vi "Configure OVP.vi"(7 "Enable OVP (T: Enable)":bool=TRUE, 8 "error in (no error)":errorcluster, 9 "Voltage Limit (6.5 V)":dbl=6.5 format="%.2f", 10 "Channel (0: 30V Channel)":T1 caption="Channel (0: +6V)" items=["30V/3A Channel", "30V/3A Channel", "5V/3A Channel"], 11 "VISA resource name":refnum<visa-resource-name>) -> (0 "error out":errorcluster, 3 "VISA resource name out":refnum<visa-resource-name>)   [LabVIEW 2020, in "RIGOL DP800 Series.lvlib"]
doc: "Configures over voltage protection (OVP) of the power supply. Specify the voltage limit and whether to enable or disable OVP."
uses:
  <instrlib>/RIGOL DP800 Series/RIGOL DP800 Series.lvlib
  <instrlib>/RIGOL DP800 Series/Public/Channels.ctl
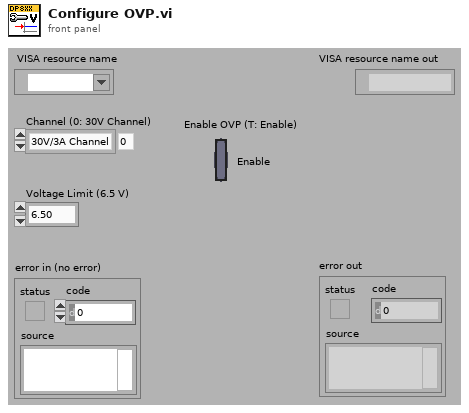
[diagram p1: front panel]
types:
  T1 = typedef "RIGOL DP800 Series.lvlib/Channels.ctl" = i32
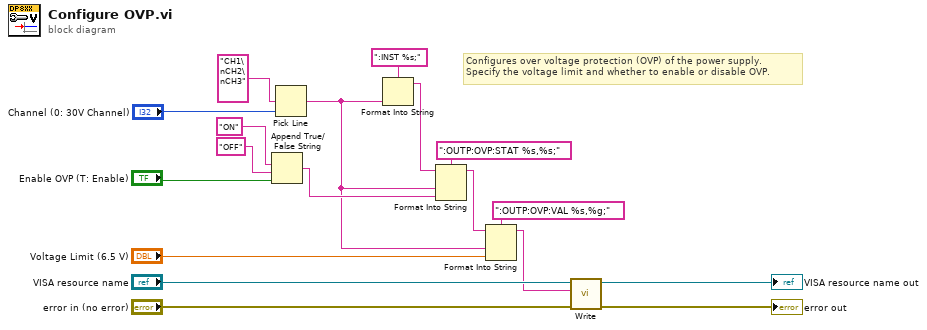
[diagram p0: block diagram]
diagram:
  # "Configures over voltage protection (OVP) of the power supply.  \nSpecify the voltage limit and whether to enable or disable OVP."
  n1 = Append True/False String(1:"Enable OVP (T: Enable)", 2:"OFF", 3:"ON") -> (0:w13:string)  [unwired: 1 out]
  n2 = Pick Line(multi-line string="CH1\nCH2\nCH3", line index="Channel (0: 30V Channel)") -> (output string=w8:string)  [unwired: 1 out]
  n3 = Format Into String(format string=":INST %s;", w8) -> (resulting string=w7:string)  [unwired: 2 in, 1 out]
  n4 = Format Into String(format string=":OUTP:OVP:STAT %s,%s;", initial string=w7, w8, w13) -> (resulting string=w12:string)  [unwired: 1 in, 1 out]
  n5 = Format Into String(format string=":OUTP:OVP:VAL %s,%g;", initial string=w12, w8, "Voltage Limit (6.5 V)") -> (resulting string=w2:string)  [unwired: 1 in, 1 out]
  n6 = call <instrlib>:"Write.vi"("error in (no error)"="error in (no error)", "Write Buffer (\"\")"=w2, "VISA resource name"="VISA resource name") -> ("error out"=→"error out":errorcluster, "VISA resource name out"=→"VISA resource name out":refnum<visa-resource-name>)  [unwired: 7 in]
